vi "Prueba_mqtt.vi"() -> ()   [LabVIEW 2025]
panel:
  out "Numeric":i32
  out "error out":errorcluster
  in  "stop":bool
  out "Lectura MQTT":string
  in  "TOPIC":string
  in  "IP":string
  in  "VISA resource name":refnum<visa-resource-name>
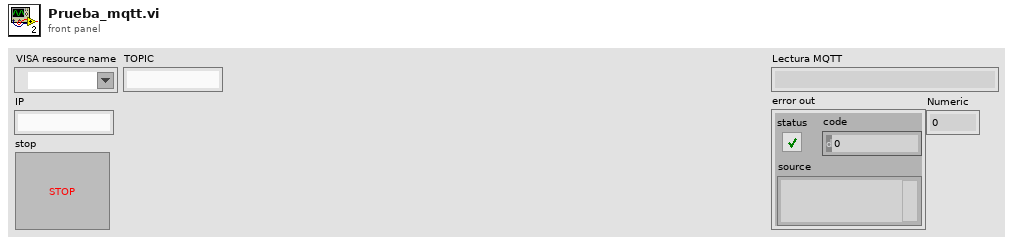
[diagram p1: front panel]
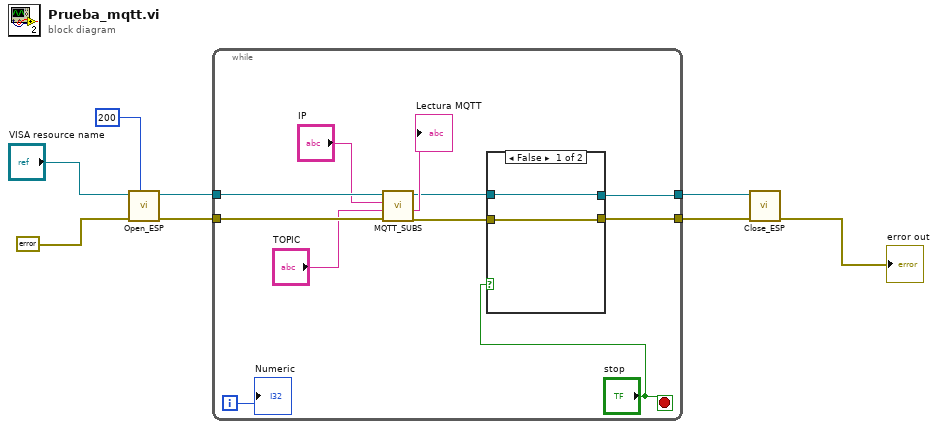
[diagram p0: block diagram]
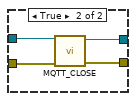
[diagram p2: hidden frame]
diagram:
  n1 = call "Open_ESP.vi"("timeout (10sec)"=u32 200, "error in (no error)"=errorcluster {"status"=FALSE, "code"=0, "source"=""}, "VISA resource name"="VISA resource name") -> ("error out"=w5:errorcluster, "VISA resource name out"=w6:refnum<visa-resource-name>)  [unwired: 7 in]
  n2 = while {
    tunnel: w5 -> [w18]
    tunnel: [w12] -> w7
    tunnel: w6 -> [w19]
    tunnel: [w13] -> w8
    i -> [w14]
    stop <- "stop" stop-if-true
    n3 = call "MQTT_SUBS.vi"("error in (no error)"=w18, "TOPIC"="TOPIC", "IP"="IP", "VISA resource name"=w19) -> ("error out"=w11:errorcluster, "Lectura MQTT"=→"Lectura MQTT":string, "VISA resource name out"=w10:refnum<visa-resource-name>)  [unwired: 5 in]
    n4 = case shown="False" "stop" {
      tunnel: [w21 w25] -> w13
      tunnel: [w20 w24] -> w12
      tunnel: w11 -> [w20 w23]
      tunnel: w10 -> [w21 w22]
      frame False {
      }
      frame True {
        n5 = call "MQTT_CLOSE.vi"("error in (no error)"=w23, "VISA resource name"=w22) -> ("error out"=w24:errorcluster, "VISA resource name out"=w25:refnum<visa-resource-name>)  [unwired: 8 in]
      }
    }
    "Numeric" <- w14
  }
  n6 = call "Close_ESP.vi"("error in (no error)"=w7, "VISA resource name"=w8) -> ("error out"=→"error out":errorcluster)  [unwired: 9 in]
